vi "loops_queue.vi"() -> ()   [LabVIEW 2022 SP3]
panel:
  in  "Stop":bool
  out "millisecond timer value 2":u32
  out "millisecond timer value":u32
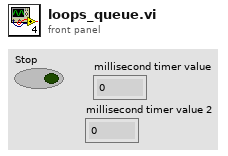
[diagram p1: front panel]
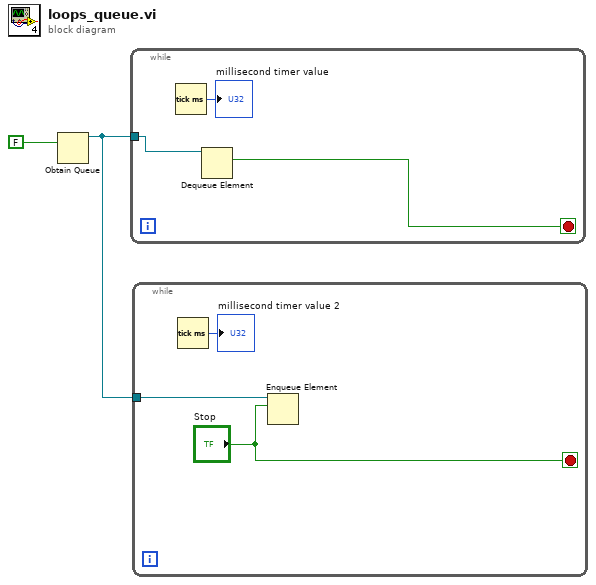
[diagram p0: block diagram]
diagram:
  n1 = Obtain Queue(element data type=FALSE) -> (queue out=w1:refnum<queue>)  [unwired: 4 in, 2 out]
  n2 = while {
    tunnel: w1 -> [w4]
    stop <- w3 stop-if-true
    n3 = Tick Count (ms)() -> (millisecond timer value=→"millisecond timer value":u32)
    n4 = Dequeue Element(queue=w4) -> (element=w3:bool)  [unwired: 2 in, 3 out]
  }
  n5 = while {
    tunnel: w1 -> [w7]
    stop <- "Stop" stop-if-true
    n6 = Tick Count (ms)() -> (millisecond timer value=→"millisecond timer value 2":u32)
    n7 = Enqueue Element(queue=w7, element="Stop") -> ()  [unwired: 2 in, 3 out]
  }
